vi "InsertPoweV.vi"(8 "error in":errorcluster) -> (0 "error out":errorcluster)   [LabVIEW 2014, in "DataBase.lvlib"]
uses:
  <vilib>/addons/database/Connection.llb/DB Tools Open Connec (String).vi
  <vilib>/addons/database/Connection.llb/Conn Execute.vi
  <vilib>/addons/database/Recordset.llb/Rec Destroy - Connection.vi
  DataBase.lvlib
  <vilib>/addons/database/NI_Database_API.lvlib
panel:
  in  "电压":T1
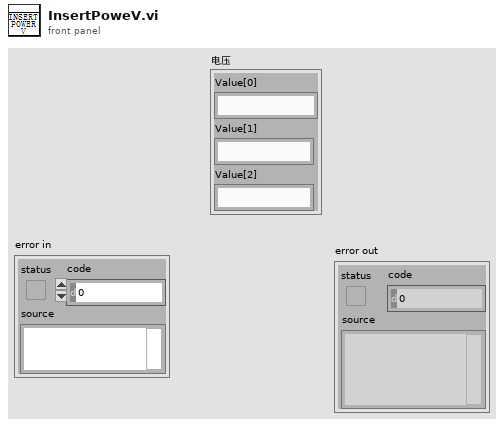
[diagram p1: front panel]
types:
  T1 = cluster{"Value[0]":string, "Value[1]":string, "Value[2]":string}
  T2 = typedef "NI_Database_API.lvlib/Conn ObjectReference.ctl" = refnum<k1>
  T3 = typedef "NI_Database_API.lvlib/Rec ObjectReference.ctl" = refnum<k1>
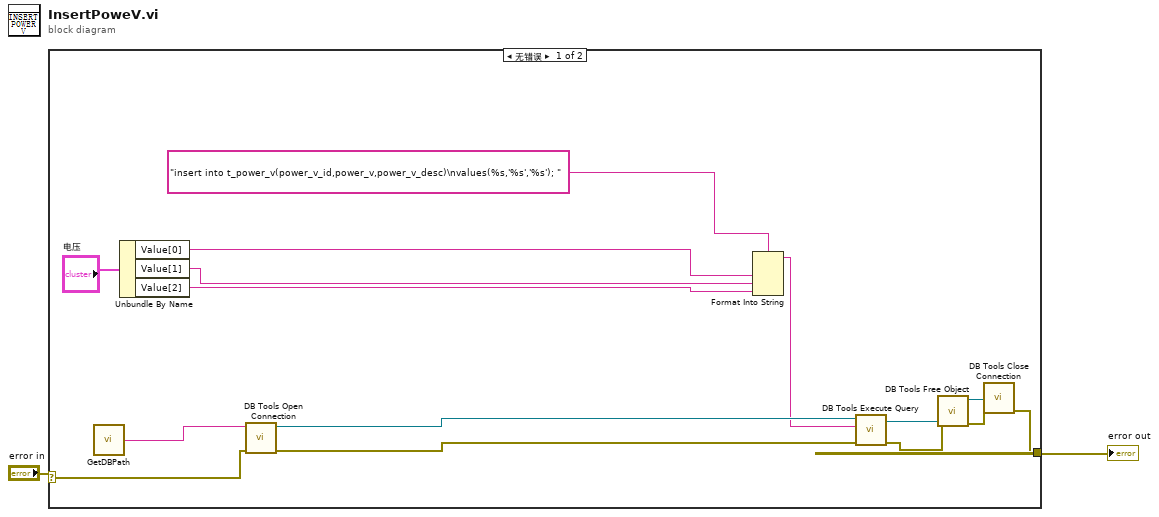
[diagram p0: block diagram]
diagram:
  n1 = case shown="无错误" "error in" {
    selector: "error in" -> [w13 w18]
    tunnel: [w12 w18] -> w1
    frame No Error {
      n2 = call "GetDBPath.vi"() -> ("Connection"=w11:string)  [unwired: 1 in]
      n3 = Unbundle By Name("电压") -> ("Value[0]"=w6:string, "Value[1]"=w7:string, "Value[2]"=w8:string)
      n4 = call-poly <vilib>:"DB Tools Open Connection.vi"("error in (no error)"=w13, "connection information"=w11) -> ("error out"=w16:errorcluster, "connection reference"=w17:T2)  [unwired: 6 in]
      n5 = Format Into String(format string="insert into t_power_v(power_v_id,power_v,power_v_desc)\nvalues(%s,'%s','%s'); ", w6, w7, w8) -> (resulting string=w3:string)  [unwired: 2 in, 1 out]
      n6 = call-poly <vilib>:"DB Tools Execute Query.vi"("error in (no error)"=w16, "SQL query"=w3, "connection reference"=w17) -> ("error out"=w9:errorcluster, "recordset reference"=w10:T3)  [unwired: 5 in]
      n7 = call-poly <vilib>:"DB Tools Free Object.vi"("error in (no error)"=w9, "recordset reference"=w10) -> ("error out"=w15:errorcluster, "connection reference"=w14:T2)  [unwired: 8 in]
      n8 = call <vilib>:"DB Tools Close Connection.vi"("error in (no error)"=w15, "connection reference"=w14) -> ("error out"=w12:errorcluster)  [unwired: 5 in]
    }
    frame Error {
    }
  }
  "error out" <- w1
